vi "Thingview.vi"(0 "value":dbl) -> ()   [LabVIEW 2023]
uses:
  <vilib>/httpClient/LabVIEWHTTPClient.lvlib
panel:
  in  "Thing View URL":string
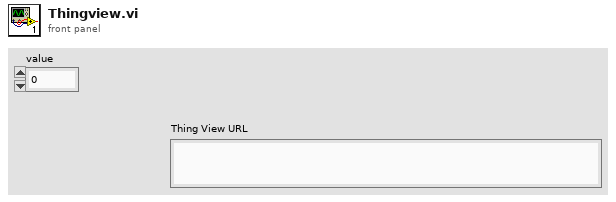
[diagram p1: front panel]
types:
  T1 = typedef "LabVIEWHTTPClient.lvlib/ClientHandle.ctl" = refnum<k1>
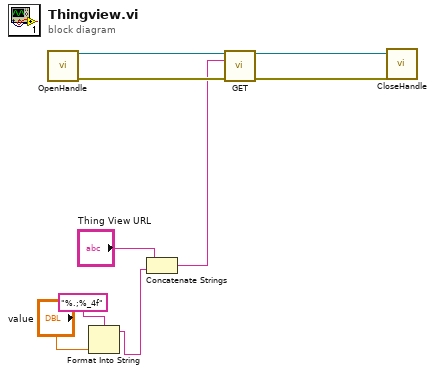
[diagram p0: block diagram]
diagram:
  n1 = call <vilib>:"OpenHandle.vi"() -> ("client handle out"=w9:T1, "error out"=w7:errorcluster)  [unwired: 14 in]
  n2 = Format Into String(format string="%.;%_4f", "value") -> (resulting string=w4:string)  [unwired: 2 in, 1 out]
  n3 = Concatenate Strings("Thing View URL", w4) -> (w1:string)
  n4 = call <vilib>:"GET.vi"("client handle"=w9, "url"=w1, "error in (no error)"=w7) -> ("client handle out"=w8:T1, "error out"=w6:errorcluster)  [unwired: 9 in, 2 out]
  n5 = call <vilib>:"CloseHandle.vi"("client handle"=w8, "error in (no error)"=w6) -> ()  [unwired: 13 in, 1 out]
